vi "DSF.Engine.Transceiver Thread.Transfer.Build.vi"(8 "error in (no error)":errorcluster, 10 "Transfer":refnum<class "DSF.Engine.Transfer.lvclass">, 11 "Transceiver Thread in":refnum<class "DSF.Engine.Transceiver Thread.lvclass">) -> (0 "error out":errorcluster, 3 "Transceiver Thread out":refnum<class "DSF.Engine.Transceiver Thread.lvclass">)   [LabVIEW 2017, in "Data Sharing Framework Engine.lvlib" / "DSF.Engine.Transceiver Thread.lvclass"]
uses:
  DSF.Engine.Transceiver Thread.lvclass
  Transfer/DSF.Engine.Transfer.lvclass
  Transfer/DSF.Engine.Transfer.lvclass/DSF.Engine.Transfer.ctl
  DSF.Engine.Transceiver Thread.lvclass/DSF.Engine.Transceiver Thread.ctl
  Pointer/DSF.Engine.Pointer.DBL.lvclass/DSF.Engine.Pointer.DBL.ctl
  <vilib>/National Instruments/Memory Manager/Classes/Pointer/Memory.Pointer.lvclass/Memory.Pointer.ctl
  Pointer/DSF.Engine.Pointer.DBL.Get Channel Count.vi
  <vilib>/National Instruments/Memory Manager/Classes/Pointer/Memory.Pointer.Read.vi
  <vilib>/National Instruments/Memory Manager/Classes/Pointer/Memory.Pointer.Read.1D.DBL.vi
  <vilib>/National Instruments/Memory Manager/Classes/Pointer/Memory.Pointer.Read.No Check.1D.DBL.vi
  <vilib>/National Instruments/Memory Manager/Classes/Pointer/Memory.Pointer.Parameter Check.Null Pointer.vi
  <vilib>/National Instruments/Memory Manager/Classes/Pointer/Memory.Pointer.Parameter Check.Subset.Power of 2.vi
  <vilib>/National Instruments/Memory Manager/Classes/Pointer/Memory.Pointer.Get Address.vi
  <vilib>/National Instruments/Memory Manager/Classes/Pointer/Memory.Pointer.Errors.vi
  <vilib>/National Instruments/Memory Manager/Classes/Pointer/Memory.Pointer.Errors.Null Pointer.vi
  <vilib>/National Instruments/Memory Manager/Classes/Pointer/Memory.Pointer.Errors.Out of Bounds.vi
  <vilib>/National Instruments/Memory Manager/Classes/Pointer/Memory.Pointer.Get Size.vi
  <vilib>/National Instruments/Memory Manager/Classes/Pointer/Memory.Pointer.Count to Size.Power of 2.vi
  <vilib>/National Instruments/Memory Manager/Classes/Pointer/Memory.Pointer.Errors.Create Error.vi
  <vilib>/NI/Static Error Handling/VIs/Static Error Handling.Source Buffer.Write.String.vi
  <vilib>/National Instruments/Memory Manager/Classes/Pointer/Memory.Pointer.Errors.Write Pointer Size.vi
  <vilib>/NI/Static Error Handling/VIs/Static Error Handling.Source Buffer.Write.Numeric.Scalar.Base10.vi
  <vilib>/NI/Static Error Handling/VIs/Static Error Handling.Source Buffer.Write.Numeric.Scalar.Base10 (U64).vi
  <vilib>/NI/Static Error Handling/VIs/Static Error Handling.Error Cluster Constant.vi
  <vilib>/NI/Static Error Handling/VIs/Static Error Handling.Error Cluster Constant (512B).vi
  <vilib>/NI/Static Error Handling/VIs/Static Error Handling.Parameters.Status.Set.vi
  <vilib>/NI/Static Error Handling/VIs/Static Error Handling.Parameters.Code.Set.vi
  <vilib>/NI/Static Error Handling/VIs/Static Error Handling.Parameters.VI Source.Set.vi
  <vilib>/National Instruments/Memory Manager/Constants/Memory.Constants.vi
  <vilib>/National Instruments/Memory Manager/Constants/Memory.Constants.Library Name.vi
  <vilib>/National Instruments/Memory Manager/Classes/Pointer/Memory.Pointer.Errors.Get Info.vi
  Pointer/DSF.Engine.Pointer.DBL.lvclass
  C:/Program Files (x86)/National Instruments/LabVIEW 2017/vi.lib/National Instruments/Memory Manager/Classes/Pointer/Memory.Pointer.lvclass
  Buffer/DSF.Engine.Memory.Buffer.Write.vi
  Buffer/DSF.Engine.Memory.Buffer.Write.1D.U64.vi
  Buffer/DSF.Engine.Memory.Buffer.Write.1D.U32.vi
  Buffer/DSF.Engine.Memory.Buffer.Write.1D.U16.vi
  Buffer/DSF.Engine.Memory.Buffer.Write.1D.U8.vi
  Buffer/DSF.Engine.Memory.Buffer.Write.1D.I64.vi
  Buffer/DSF.Engine.Memory.Buffer.Write.1D.I32.vi
  Buffer/DSF.Engine.Memory.Buffer.Write.1D.I16.vi
  Buffer/DSF.Engine.Memory.Buffer.Write.1D.I8.vi
  Buffer/DSF.Engine.Memory.Buffer.Write.1D.DBL.vi
  Buffer/DSF.Engine.Memory.Buffer.Write.1D.SGL.vi
  Buffer/DSF.Engine.Memory.Buffer.Write.1D.Bool.vi
  Buffer/DSF.Engine.Memory.Buffer.lvclass
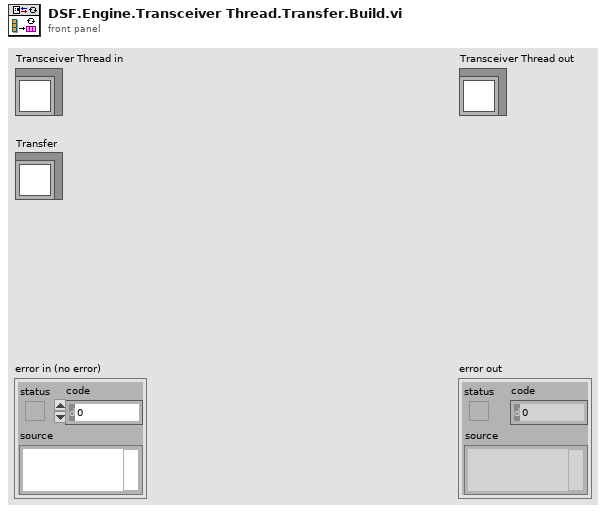
[diagram p1: front panel]
types:
  T1 = typedef "Data Sharing Framework Engine.lvlib/DSF Runtime Channel Block.ctl" = cluster{"data type":T2, "count":u64, "buffer offset":u64}
  T2 = typedef "DSF Configuration API.lvlib/DSF Data Type.ctl" = enum8{"Bool", "SGL", "DBL", "I8", "I16", "I32", "I64", "U8", "U16", "U32", "U64"}
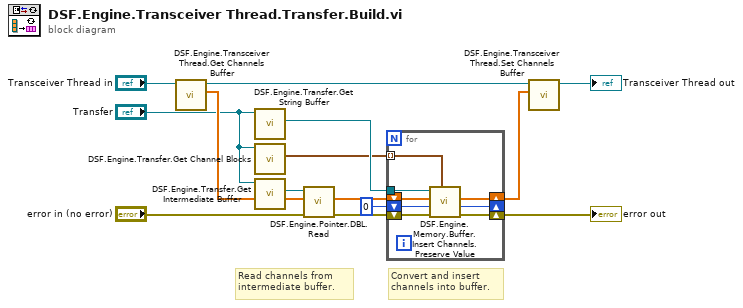
[diagram p0: block diagram]
diagram:
  # "Convert and insert channels into buffer."
  # "Read channels from intermediate buffer."
  n1 = call "DSF.Engine.Transceiver Thread.Get Channels Buffer.vi"("Transceiver Thread in"="Transceiver Thread in") -> ("channels buffer"=w7:dbl[], "Transceiver Thread out"=w5:refnum<class "DSF.Engine.Transceiver Thread.lvclass">)  [unwired: 9 in]
  n2 = call "DSF.Engine.Transfer.Get String Buffer.vi"("Transfer in"="Transfer") -> ("Buffer"=w13:refnum<class "DSF.Engine.Memory.Buffer.lvclass">)  [unwired: 9 in, 1 out]
  n3 = call "DSF.Engine.Transfer.Get Channel Blocks.vi"("Transfer in"="Transfer") -> ("channel blocks"=w2:T1[])  [unwired: 9 in, 1 out]
  n4 = call "DSF.Engine.Transfer.Get Intermediate Buffer.vi"("Transfer in"="Transfer") -> ("DBL Buffer"=w12:refnum<class "DSF.Engine.Pointer.DBL.lvclass">)  [unwired: 9 in, 1 out]
  n5 = call "DSF.Engine.Pointer.DBL.Read.vi"("error in (no error)"="error in (no error)", "buffer in"=w7, "DBL Pointer in"=w12) -> ("error out"=w9:errorcluster, "buffer out"=w10:dbl[])  [unwired: 6 in, 1 out]
  n6 = for {
    shift-right: [w20] -> w6
    shift-left: w10 -> [w21]
    shift-right: [w19] -> w14
    shift-left: w9 -> [w22]
    tunnel: w13 -> [w18]
    tunnel: w2 -> [w17] mode=indexing
    shift-right: [w16] -> _
    shift-left: u64 0 ("channels buffer index in") -> [w15]
    n7 = call "DSF.Engine.Memory.Buffer.Insert Channels.Preserve Value.vi"("channel block"=w17, "error in (no error)"=w22, "channels buffer index in"=w15, "channels buffer in"=w21, "Buffer in"=w18) -> ("error out"=w19:errorcluster, "channels buffer index out"=w16:u64, "channels buffer out"=w20:dbl[])  [unwired: 3 in, 1 out]
  }
  "error out" <- w14
  n8 = call "DSF.Engine.Transceiver Thread.Set Channels Buffer.vi"("channels buffer"=w6, "Transceiver Thread in"=w5) -> ("Transceiver Thread out"=→"Transceiver Thread out":refnum<class "DSF.Engine.Transceiver Thread.lvclass">)  [unwired: 9 in]
